vi "CombU16toU32.vi"(1 "数据高16位":u32 format="%x", 2 "数据低16位":u32 format="%x") -> (0 "32位数据输出":u32 format="%x")   [LabVIEW 2015]
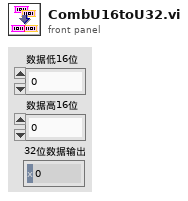
[diagram p1: front panel]
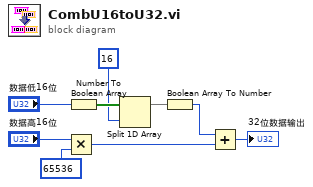
[diagram p0: block diagram]
diagram:
  n1 = Multiply(x="数据高16位", y=65536) -> (x*y=w1:u32)
  n2 = Number To Boolean Array(number="数据低16位") -> (Boolean array=w9:bool[])
  n3 = Split 1D Array(array=w9, index=16) -> (first subarray=w6:bool[])  [unwired: 1 out]
  n4 = Boolean Array To Number(Boolean array=w6) -> (number=w5:u32)
  n5 = Add(x=w5, y=w1) -> (x+y=→"32位数据输出":u32)
